vi "Error Code Dialog.vi"(8 "error in":errorcluster, 11 "Selection":T1) -> (0 "error out":errorcluster, 1 "Cancel Out":bool, 3 "Error VI Path":path)   [LabVIEW 2020, in "ConstantErrorsMaker.lvlib"]
uses:
  ConstantErrorsMaker.lvlib
  Continue.ctl
  MulticolumListbox.ctl
  Selection Info--cluster.ctl
  Selection Type--enum.ctl
panel:
  in  "Information":string="These are the benefits of having Error Constant VIs\n\n1. Centralized Error Management:\n   - Single Point of Editing: by storing error codes and descriptions in constants, you can modify them in one place, ensuring consistency across the entire application. This streamlines maintenance and avoids potential errors due to inconsistencies.\n   - Enhanced Organization: Grouping error-related information in constants improves code readability and understanding. It also makes it easier to quickly locate and update error-related logic.\n\n2. Improved Code Readability:\n   - Clearer Meaning: Instead of using raw error codes directly in code, constants provide meaningful names for errors, making code more self-explanatory and easier for others to comprehend.\n   - Reduced Redundancy: Constants eliminate the need to repeatedly define error codes and descriptions throughout the code, reducing redundancy and improving code maintainability.\n\n3. Error Tracking and Debugging:\n   - Identifying Error Sources: By using constant VIs, you can easily track where specific errors are being generated within the application. This aids in debugging and pinpointing the root causes of issues.\n   - Debugging Efficiency: Constants make it easier to search for error-related code and analyze error handling logic, facilitating debugging and problem resolution.\n\n4. Flexibility for Customization:\n   - Adaptability: If error codes or descriptions need to change, you can easily update them in the constant VIs without having to modify code in multiple locations. This allows for quick adjustments and customization as needed.\n\nRanges of Custom Error Codes defined by NI:\n     –8999  through –8000\n       5000  through   9999\n  500,000  through 599,999\n"
  in  "Error Description":string
  in  "Current Error VIs Values":T3
  in  "Error Name (do not add --error.vi)":string
  in  "Continue":T4
  in  "Cancel":bool
  in  "Error Code":i32
  # "TIP: Doble click to open --error.vi Block Diagram"
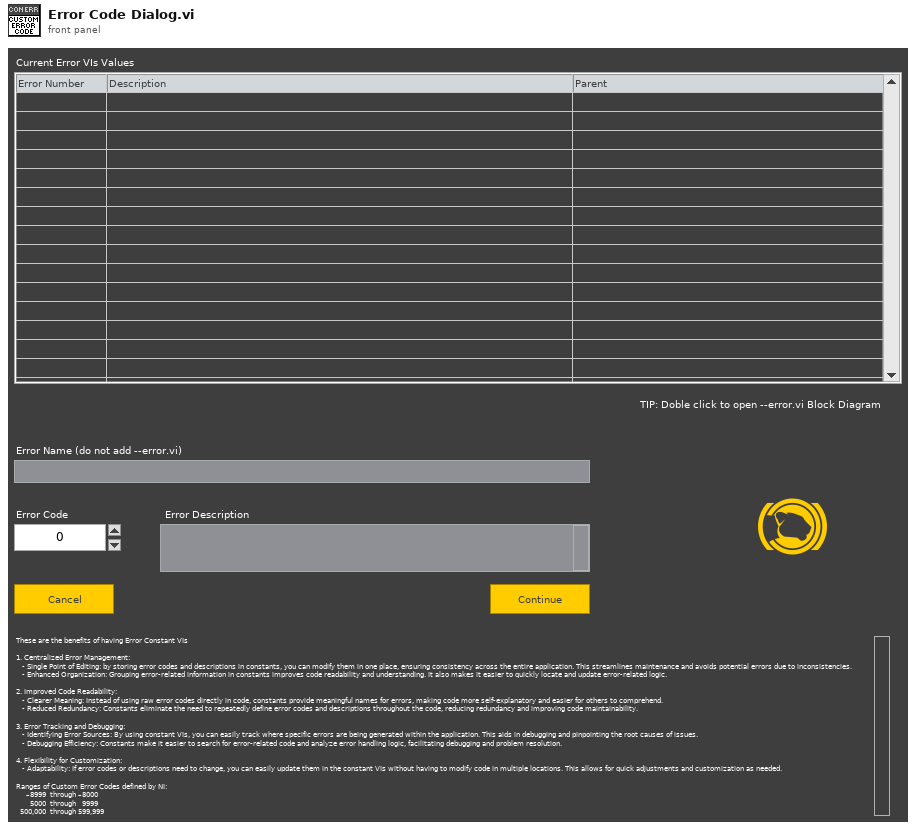
[diagram p1: front panel]
types:
  T1 = typedef "ConstantErrorsMaker.lvlib/Selection Info--cluster.ctl" = cluster{"Name":string, "Library Ref":refnum<vi>, "Application Instance":refnum<vi>, "Selection Owning Folder":path, "Selection Type":T2, "Project Reference":refnum<vi>, "LVClassLibrary Refnum":refnum<vi>}
  T2 = typedef "ConstantErrorsMaker.lvlib/Selection Type--enum.ctl" = enum16{"Project", "Library", "Class", "DQMH Singleton", "DQMH Cloneable"}
  T3 = typedef "ConstantErrorsMaker.lvlib/MulticolumListbox.ctl" = i32
  T4 = typedef "ConstantErrorsMaker.lvlib/Continue.ctl" = bool
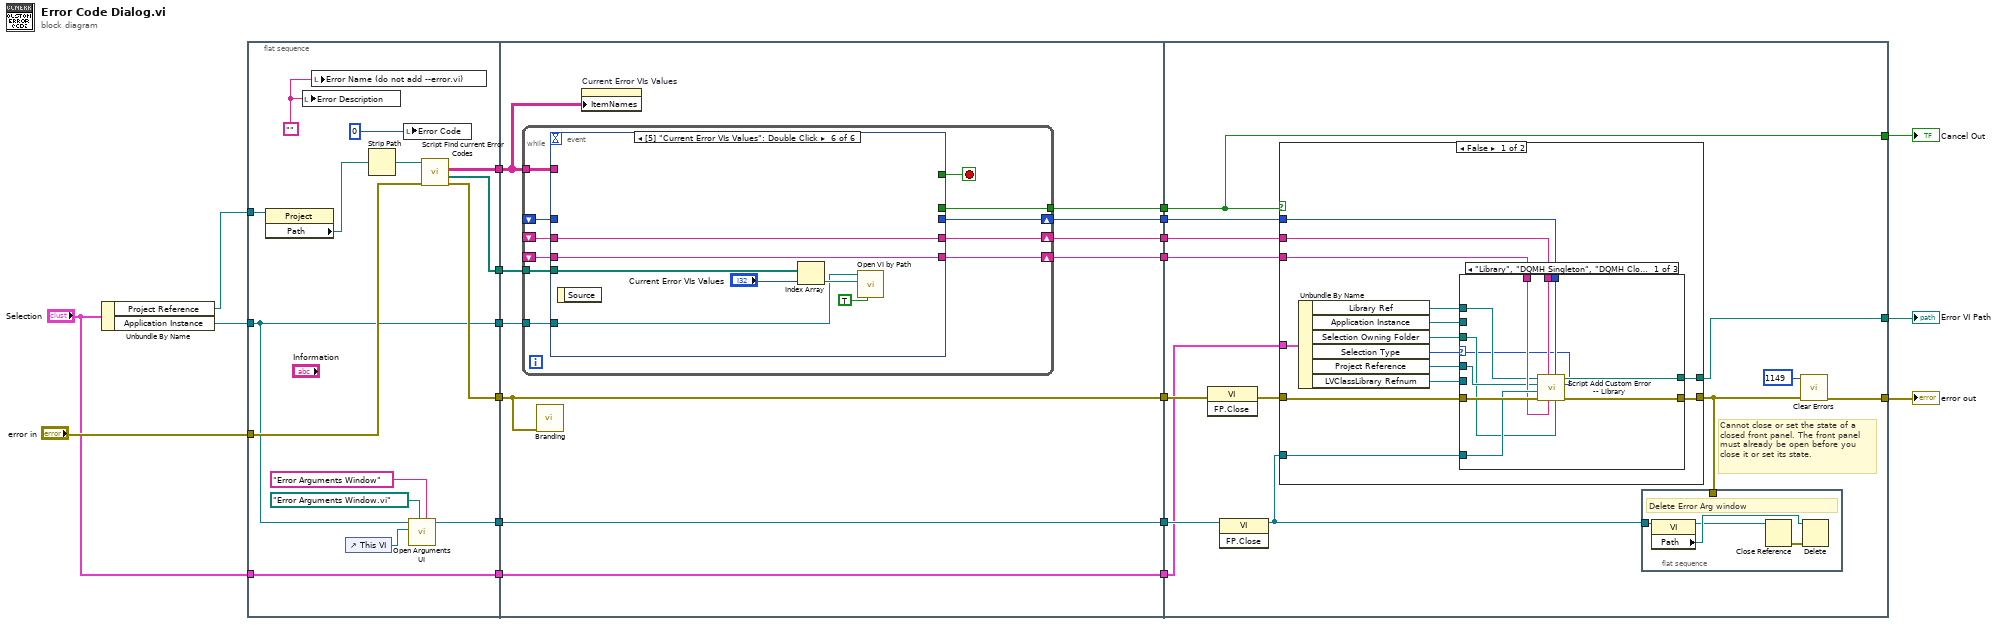
[diagram p0: block diagram]
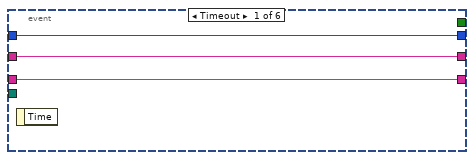
[diagram p2: hidden frame]
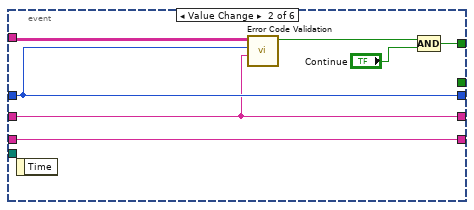
[diagram p3: hidden frame]
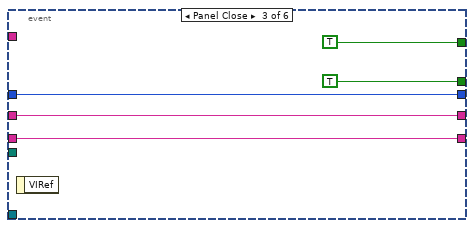
[diagram p4: hidden frame]
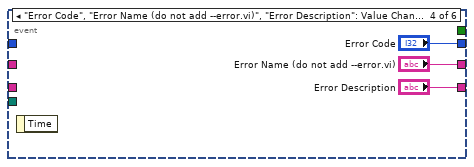
[diagram p5: hidden frame]
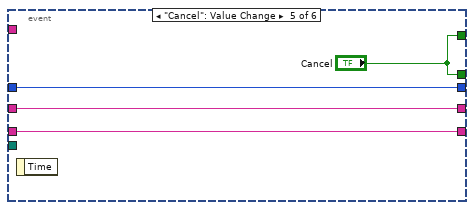
[diagram p6: hidden frame]
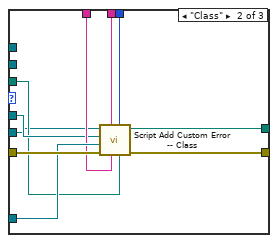
[diagram p7: hidden frame]
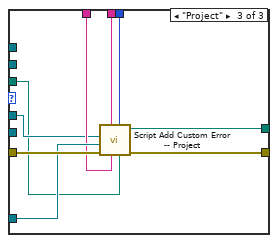
[diagram p8: hidden frame]
diagram:
  n1 = Unbundle By Name("Selection") -> ("Project Reference"=w5:refnum<vi>, "Application Instance"=w6:refnum<vi>)
  n2 = flat-sequence {
    tunnel: "error in" -> [w35]
    tunnel: [w34] -> w20
    tunnel: [w32] -> w14
    tunnel: [w30] -> w12
    tunnel: w6 -> [w25]
    tunnel: [w26] -> w8
    tunnel: [w25] -> w7
    tunnel: w5 -> [w23]
    tunnel: "Selection" -> [w24]
    tunnel: [w24] -> w3
    tunnel: w20 -> [w41]
    tunnel: [w41] -> w19
    tunnel: [w42] -> w17
    tunnel: [w45] -> w16
    tunnel: [w44] -> w15
    tunnel: w14 -> [w40]
    tunnel: [w36] -> w13
    tunnel: w12 -> [w36]
    tunnel: [w43] -> w11
    tunnel: w8 -> [w39]
    tunnel: w7 -> [w38]
    tunnel: w3 -> [w37]
    tunnel: [w37] -> w2
    tunnel: [w98] -> w9
    tunnel: w19 -> [w95]
    tunnel: w17 -> [w88]
    tunnel: w16 -> [w94]
    tunnel: w15 -> [w93]
    tunnel: w13 -> [w91]
    tunnel: w11 -> [w89]
    tunnel: [w88] -> w10
    tunnel: w2 -> [w87]
    tunnel: [w86] -> w1
    frame #0 {
      w27 = "" ("Error Message")
      n3 = property class="Project"(reference=w23) -> ("Path"=w22:path)  [unwired: 1 in, 2 out]
      n4 = local write "Error Description"(w27) -> ()
      n5 = local write "Error Name (do not add --error.vi)"(w27) -> ()
      n6 = control-ref of="This VI"() -> (w31:refnum<vi>)
      n7 = Strip Path(path=w22) -> (stripped path=w21:path)  [unwired: 1 out]
      n8 = local write "Error Code"(0 ("Error Code")) -> ()
      n9 = call "Open Arguments UI.vi"("Title"="Error Arguments Window", "Path"=path "Error Arguments Window.vi", "Calling VI Ref"=w31, "App Instance"=w25) -> ("Error Arguments Window Ref"=w30:refnum<vi>)  [unwired: 6 in, 1 out]
      n10 = call "Script Find current Error Codes.vi"("error in"=w35, "Selection Owning Folder"=w21) -> ("error out"=w34:errorcluster, "All Error VIS"=w26:path[], "Error and Descriptions Table"=w32:string[][])  [unwired: 7 in]
    }
    frame #1 {
      n11 = while {
        shift-right: [w55] -> w44
        shift-left: _ -> [w54]
        shift-right: [w53] -> w45
        shift-left: _ -> [w52]
        tunnel: [w51] -> w42
        tunnel: w40 -> [w50]
        shift-right: [w49] -> w43
        shift-left: _ -> [w48]
        tunnel: w39 -> [w47]
        tunnel: w38 -> [w46]
        stop <- w56 stop-if-true
        n12 = event shown="[5] \"Current Error VIs Values\": Double Click" {
          selector: _ -> [_ _ _ _ _ _]
          dyn-events: _ -> [_ _ _ _ _ _]
          timeout: _ -> [_ _ _ _ _ _]
          tunnel: [_ w65 TRUE ("Cancel") _ "Cancel" _] -> w56
          tunnel: [w59 w66 w67 "Error Code" w77 _] -> w55
          tunnel: w54 -> [w59 w66 w67 _ w77 _]
          tunnel: [w58 w60 w71 "Error Name (do not add --error.vi)" w78 w85] -> w53
          tunnel: w52 -> [w58 w60 w71 _ w78 w85]
          tunnel: [_ _ TRUE ("Cancel") _ "Cancel" _] -> w51
          tunnel: w50 -> [_ w62 _ _ _ _]
          tunnel: [w57 w61 w68 "Error Description" w75 w84] -> w49
          tunnel: w48 -> [w57 w61 w68 _ w75 w84]
          tunnel: w47 -> [_ _ _ _ _ w83]
          tunnel: w46 -> [_ _ _ _ _ w80]
          event Timeout {
            n13 = event-data() -> ()  [unwired: 1 in, 1 out]
          }
          event Value Change {
            n14 = event-data() -> ()  [unwired: 1 in, 1 out]
            n15 = call "Error Code Validation.vi"("Error Name"=w60, "New Error Code"=w66, "Error Codes and Descriptions"=w62) -> ("Continue"=w63:bool)  [unwired: 8 in]
            n16 = Compound Arithmetic op=AND(w63, "Continue") -> (w65:T4)
          }
          event Panel Close {
            n17 = event-data() -> ()  [unwired: 1 in, 1 out]
          }
          event "Error Code", "Error Name (do not add --error.vi)", "Error Description": Value Change {
            n18 = event-data() -> ()  [unwired: 1 in, 1 out]
          }
          event "Cancel": Value Change {
            n19 = event-data() -> ()  [unwired: 1 in, 1 out]
          }
          event Double Click {
            n20 = event-data() -> ()  [unwired: 1 in, 1 out]
            n21 = Index Array(array=w83, index="Current Error VIs Values") -> (element=w81:path)
            n22 = call "Open VI by Path.vi"("Block Diagram?"=TRUE, "VI Path"=w81, "Application in"=w80) -> ()  [unwired: 8 in, 1 out]
          }
        }
      }
      n23 = call "Branding.vi"("error in"=w41) -> ()  [unwired: 11 in]
      n24 = property on="Current Error VIs Values" class="MCListbox (strict)"("ItemNames"=w40) -> ()  [unwired: 2 in, 2 out]
    }
    frame #2 {
      # "Cannot close or set the state of a closed front panel. The front panel must already be open before you close it or set its state."
      n25 = invoke class="VI" method="FP.Close"(error in=w95) -> (error out=w97:errorcluster)  [unwired: 2 in, 2 out]
      n26 = invoke class="VI" method="FP.Close"(reference=w91) -> (reference out=w90:refnum<vi>)  [unwired: 2 in, 2 out]
      n27 = case shown="False" w88 {
        tunnel: [w111 w147] -> w96
        tunnel: w97 -> [w116 w147]
        tunnel: w94 -> [w112 _]
        tunnel: w93 -> [w115 _]
        tunnel: w90 -> [w114 _]
        tunnel: w89 -> [w113 _]
        tunnel: w87 -> [w110 _]
        tunnel: [w103 _] -> w86
        frame False {
          n28 = Unbundle By Name(w110) -> ("Library Ref"=w109:refnum<vi>, "Application Instance"=w108:refnum<vi>, "Selection Owning Folder"=w107:path, "Selection Type"=w106:T2, "Project Reference"=w105:refnum<vi>, "LVClassLibrary Refnum"=w104:refnum<vi>)
          n29 = case shown="\"Library\", \"DQMH Singleton\", \"DQMH Cloneable\"" w106 {
            selector: w106 -> [w117 _ _]
            tunnel: w116 -> [w127 w137 w146]
            tunnel: w115 -> [w126 w136 w145]
            tunnel: w114 -> [w125 w135 w144]
            tunnel: w113 -> [w124 w134 w143]
            tunnel: w112 -> [w123 w133 w142]
            tunnel: [w122 w132 w141] -> w111
            tunnel: w109 -> [w121 _ _]
            tunnel: w108 -> [_ _ _]
            tunnel: w107 -> [w119 w130 w139]
            tunnel: w105 -> [w120 w131 w140]
            tunnel: w104 -> [_ w129 _]
            tunnel: [w118 w128 w138] -> w103
            frame "Library", "DQMH Singleton", "DQMH Cloneable" {
              n30 = call "Script Add Custom Error -- Library.vi"("Selection Type"=w117, "Selection Owning Folder"=w119, "Error Code"=w126, "Error Description"=w124, "Error Name"=w123, "error in"=w127, "Error Arguments Window Ref"=w125, "Project Reference"=w120, "Library Ref"=w121) -> ("error out"=w122:errorcluster, "Error VI Path"=w118:path)  [unwired: 1 in]
            }
            frame "Class" {
              n31 = call "Script Add Custom Error -- Class.vi"("Selection Owning Folder"=w130, "Error Code"=w136, "Error Description"=w134, "Error Name"=w133, "error in"=w137, "Error Arguments Window Ref"=w135, "Project Reference"=w131, "Class Ref"=w129) -> ("error out"=w132:errorcluster, "Error VI Path"=w128:path)  [unwired: 2 in]
            }
            frame "Project" {
              n32 = call "Script Add Custom Error -- Project.vi"("Selection Owning Folder"=w139, "Error Code"=w145, "Error Description"=w143, "Error Name"=w142, "error in"=w146, "Error Arguments Window Ref"=w144, "Project Reference"=w140) -> ("error out"=w141:errorcluster, "Error VI Path"=w138:path)  [unwired: 3 in]
            }
          }
        }
        frame True {
        }
      }
      n33 = flat-sequence {
        tunnel: w90 -> [w101]
        tunnel: w96 -> [_]
        frame #0 {
          # "Delete Error Arg window"
          n34 = property class="VI"(reference=w101) -> (reference out=w99:refnum<vi>, "Path"=w100:path)  [unwired: 1 in, 1 out]
          n35 = Close Reference(reference=w99) -> (error out=w102:errorcluster)  [unwired: 1 in]
          n36 = Delete(path (use dialog)=w100, error in=w102) -> ()  [unwired: 3 in, 3 out]
        }
      }
      n37 = call <vilib>:"Clear Errors.vi"("error in (no error)"=w96, "specific error code to clear (0: all)"=1149) -> ("error out"=w98:errorcluster)  [unwired: 4 in, 1 out]
    }
  }
  "error out" <- w9
  "Cancel Out" <- w10
  "Error VI Path" <- w1
